vi "multicolorWormSetLaserAndFilter.vi"() -> ()   [LabVIEW 2017]
panel:
  out "laserpowersuccess":bool
  in  "molecule":string(combo)="BFP"
  out "filter wheel position":u8
  out "slider position":u16
  # "MULTICOLOR WORM\nSET LASER AND FILTER APPROPRIATE FOR A SPECIFIC MOLECULE"
  # "Use this VI to set laser and filter if you want to\nacquire/display images from the camera with\nHCImageLive (the Hamamatsu camera \nsoftware)."
  # "Diagnostics"
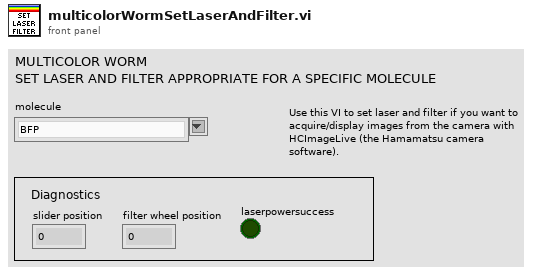
[diagram p1: front panel]
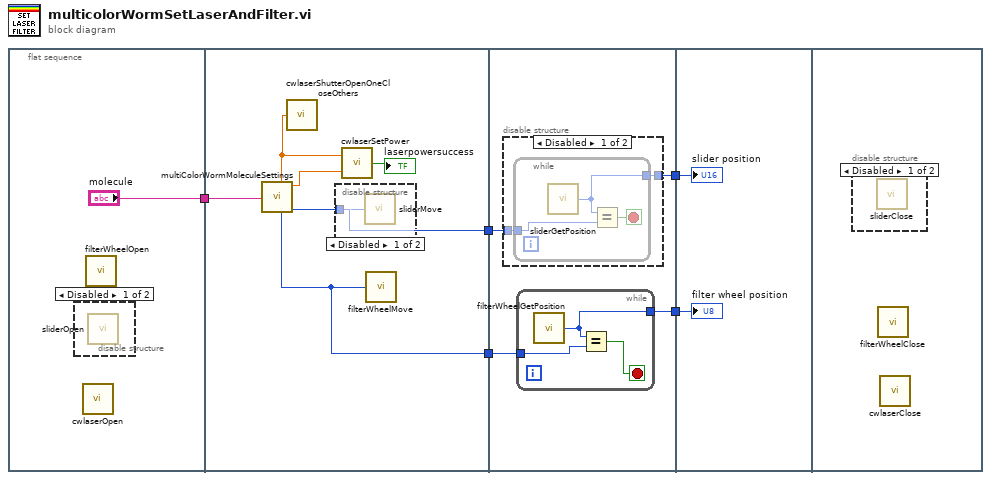
[diagram p0: block diagram]
diagram:
  n1 = flat-sequence {
    tunnel: ["molecule"] -> w1
    tunnel: [w12] -> w5
    tunnel: [w11] -> w4
    tunnel: w1 -> [w10]
    tunnel: w5 -> [w17]
    tunnel: w4 -> [w16]
    tunnel: [w15] -> w3
    tunnel: [w14] -> w2
    tunnel: w3 -> [w27]
    tunnel: w2 -> [w26]
    frame #0 {
      n2 = disable-structure shown="Disabled" {
        frame Disabled {
          n3 = call "sliderOpen.vi"() -> ()  [unwired: 2 in, 1 out]
        }
        frame Enabled {
        }
      }
      n4 = call "cwlaserOpen.vi"() -> ()  [unwired: 4 in]
      n5 = call "filterWheelOpen.vi"() -> ()  [unwired: 12 in]
    }
    frame #1 {
      n6 = call "multiColorWormMoleculeSettings.vi"("molecule"=w10) -> ("laserWavelength"=w7:dbl, "filter wheel position"=w11:u8, "laser power (mW)"=w9:dbl, "slider position"=w12:u16)  [unwired: 2 out]
      n7 = call "cwlaserShutterOpenOneCloseOthers.vi"("wavelength"=w7) -> ()  [unwired: 1 in]
      n8 = disable-structure shown="Disabled" {
        disable-tunnel: w12 -> [w13 _]
        frame Disabled {
          n9 = call "sliderMove.vi"("position"=w13) -> ()  [unwired: 1 out]
        }
        frame Enabled {
        }
      }
      n10 = call "cwlaserSetPower.vi"("power (mW)"=w9, "wavelength"=w7) -> ("success"=→"laserpowersuccess":bool)
      n11 = call "filterWheelMove.vi"("filter index"=w11) -> ()  [unwired: 1 out]
    }
    frame #2 {
      n12 = disable-structure shown="Disabled" {
        disable-tunnel: w17 -> [w19 _]
        disable-tunnel: [w18 _] -> w15
        frame Disabled {
          n13 = while {
            tunnel: w19 -> [w22]
            tunnel: [w20] -> w18
            stop <- w21 stop-if-true
            n14 = call "sliderGetPosition.vi"() -> ("position"=w20:i32)  [unwired: 1 in]
            n15 = Equal?(x=w20, y=w22) -> (x = y?=w21:bool)
          }
        }
        frame Enabled {
        }
      }
      n16 = while {
        tunnel: w16 -> [w25]
        tunnel: [w23] -> w14
        stop <- w24 stop-if-true
        n17 = call "filterWheelGetPosition.vi"() -> ("number"=w23:i32)  [unwired: 1 in]
        n18 = Equal?(x=w23, y=w25) -> (x = y?=w24:bool)
      }
    }
    frame #3 {
      "slider position" <- w27
      "filter wheel position" <- w26
    }
    frame #4 {
      n19 = disable-structure shown="Disabled" {
        frame Disabled {
          n20 = call "sliderClose.vi"() -> ()  [unwired: 2 in, 1 out]
        }
        frame Enabled {
        }
      }
      n21 = call "filterWheelClose.vi"() -> ()  [unwired: 12 in]
      n22 = call "cwlaserClose.vi"() -> ()  [unwired: 3 in]
    }
  }
